vi "niP2P Destroy Peer to Peer Stream.vi"(0 "stream session":refnum<k20>, 11 "error in (no error)":errorcluster) -> (15 "error out":errorcluster)   [LabVIEW 2010]
doc: "Unlinks the writer and reader and purges data from the stream. Any existing data in the writer is lost. If a stream is enabled, this VI disables the stream without flushing the writer before unlinking the reader and writer."
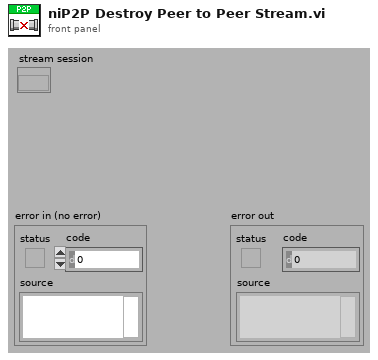
[diagram p1: front panel]
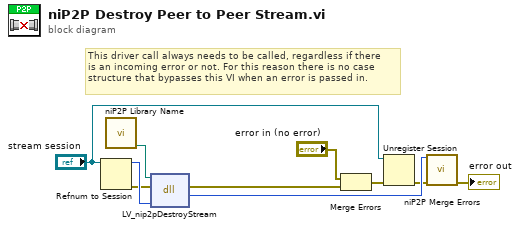
[diagram p0: block diagram]
diagram:
  # "This driver call always needs to be called, regardless if there\nis an incoming error or not. For this reason there is no case\nstructure that bypasses this VI when an error is passed in."
  n1 = Refnum to Session(7:"stream session") -> (0:w2:errorcluster, 3:w10:u64)  [unwired: 1 in]
  n2 = call <vilib>:"niP2P Library Name.vi"() -> ("nip2p libname"=w3:path)  [unwired: 10 in]
  n3 = dll-call lib="?" fn="LV_nip2pDestroyStream"(path in=w3, error in=w2, "streamHandle"=w10) -> (error out=w1:errorcluster, "return type"=w9:i32)  [unwired: 2 in, 1 out]
  n4 = Merge Errors("error in (no error)", w1) -> (w7:errorcluster)
  n5 = Unregister Session(8:w7, 11:"stream session") -> (0:w5:errorcluster)
  n6 = call <vilib>:"niP2P Merge Errors.vi"("error code"=w9, "error in"=w5) -> ("error out"=→"error out":errorcluster)  [unwired: 13 in]
